vi "Mod בחירת בדיקות עבור הממסר.vi"(0 "Enable":bool=TRUE, 5 "error in (no error)":errorcluster) -> (11 "בחר הכל":bool, 12 "בדיקת מפל מתח בין דקי הממסר תחת עומס":bool, 13 "בדיקת זמן ניתוק הממסר":bool, 14 "בדיקת זמן מיתוג הממסר":bool, 15 "בדיקת צריכת זרם של סליל הפיקוד":bool, 16 "בדיקת מתח שחרור של סליל פיקוד ללא עומס":bool, 17 "בדיקת מתח תפיסה של סליל פיקוד ללא עומס":bool, 18 "OK":bool, 19 "error out":errorcluster)   [LabVIEW 2014]
doc: "Displays a standard dialog box that prompts users to enter information, such as a user name and password.\n--------------------\n\nThis Express VI is configured as follows:\n\nMessage to Display to the User:15A בחירת בדיקות עבור הממסר\nThe inputs are: \nCheckbox: בדיקת מתח תפיסה של סליל פיקוד ללא עומס\nCheckbox: בדיקת מתח שחרור של סליל פיקוד ללא עומס\nCheckbox: בדיקת צריכת זרם של סליל הפיקוד\nCheckbox: בדיקת זמן מיתוג הממסר\nCheckbox: בדיקת זמן ניתוק הממסר\nCheckbox: בדיקת מפל מתח בין דקי הממסר תחת עומס\nCheckbox: בחר הכל"
panel:
  in  "בחר הכל":bool
  in  "בדיקת מפל מתח בין דקי הממסר תחת עומס":bool
  in  "בדיקת זמן ניתוק הממסר":bool
  in  "בדיקת זמן מיתוג הממסר":bool
  in  "בדיקת צריכת זרם של סליל הפיקוד":bool
  in  "בדיקת מתח שחרור של סליל פיקוד ללא עומס":bool
  in  "בדיקת מתח תפיסה של סליל פיקוד ללא עומס":bool
  out "String":string="15A בחירת בדיקות עבור הממסר"
  in  "Cancel":bool
  in  "OK2":bool
  in  "OK1":bool
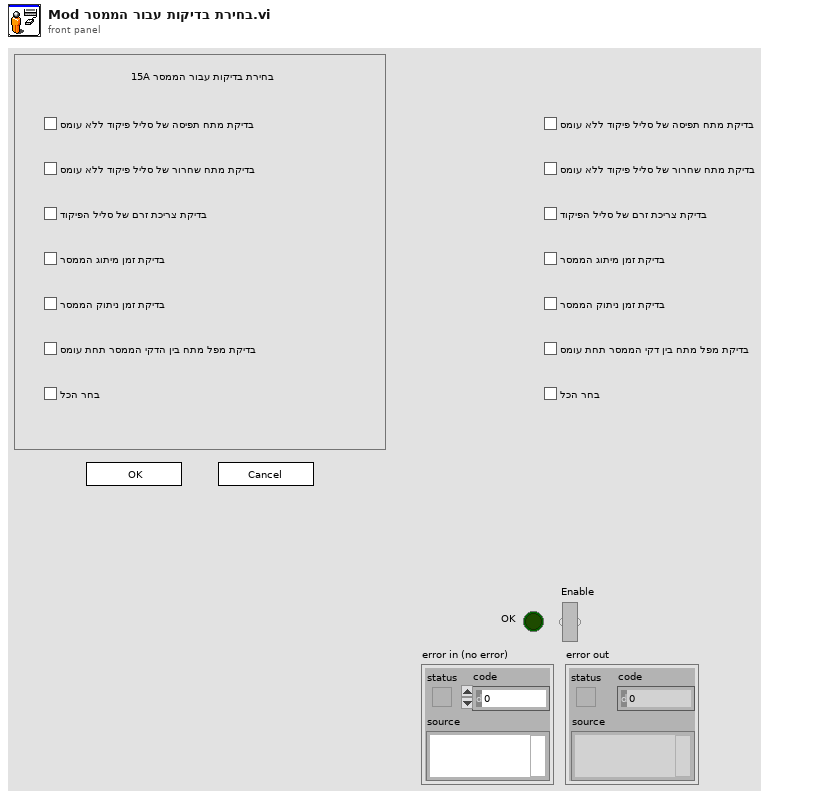
[diagram p1: front panel]
types:
  T1 = cluster{"Input Name":string, "Input Data Type":i32}[]
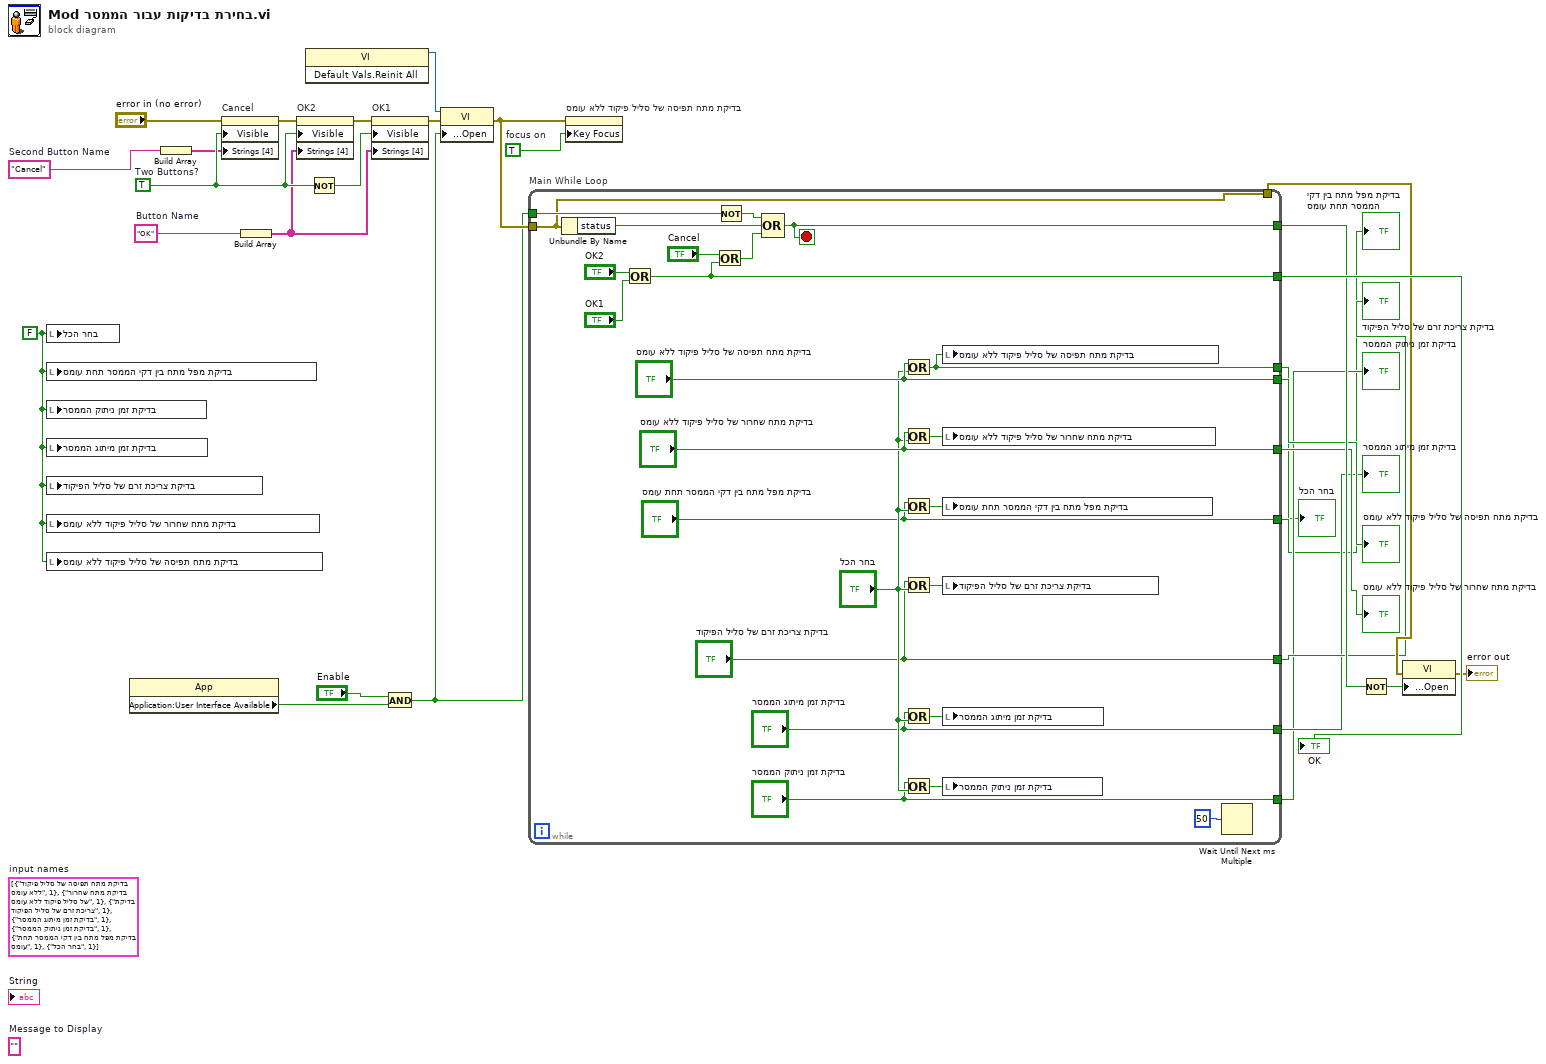
[diagram p0: block diagram]
diagram:
  w1 = FALSE ("בחר הכל")
  w8 = TRUE  # focus on
  (unwired) T1 [{"Input Name"="בדיקת מתח תפיסה של סליל פיקוד ללא עומס", "Input Data Type"=1}, {"Input Name"="בדיקת מתח שחרור של סליל פיקוד ללא עומס", "Input Data Type"=1}, {"Input Name"="בדיקת צריכת זרם של סליל הפיקוד", "Input Data Type"=1}, {"Input Name"="בדיקת זמן מיתוג הממסר", "Input Data Type"=1}, {"Input Name"="בדיקת זמן ניתוק הממסר", "Input Data Type"=1}, {"Input Name"="בדיקת מפל מתח בין דקי הממסר תחת עומס", "Input Data Type"=1}, {"Input Name"="בחר הכל", "Input Data Type"=1}]  # input names
  w21 = "Cancel"  # Second Button Name
  w19 = "OK"  # Button Name
  (unwired) ""  # Message to Display
  w29 = TRUE  # Two Buttons?
  n1 = local write "בחר הכל"(w1) -> ()
  n2 = local write "בדיקת מפל מתח בין דקי הממסר תחת עומס"(w1) -> ()
  n3 = local write "בדיקת זמן ניתוק הממסר"(w1) -> ()
  n4 = local write "בדיקת זמן מיתוג הממסר"(w1) -> ()
  n5 = local write "בדיקת צריכת זרם של סליל הפיקוד"(w1) -> ()
  n6 = local write "בדיקת מתח שחרור של סליל פיקוד ללא עומס"(w1) -> ()
  n7 = local write "בדיקת מתח תפיסה של סליל פיקוד ללא עומס"(w1) -> ()
  n8 = property class="App"() -> ("Application:User Interface Available"=w11:bool)  [unwired: 2 in, 2 out]
  n9 = Build Array(w21) -> (w22:string[])
  n10 = property on="Cancel" class="Bool"(error in="error in (no error)", "Visible"=w29, "Strings [4]"=w22) -> (error out=w26:errorcluster)  [unwired: 1 in, 1 out]
  n11 = Build Array(w19) -> (w20:string[])
  n12 = property on="OK2" class="Bool"(error in=w26, "Visible"=w29, "Strings [4]"=w20) -> (error out=w25:errorcluster)  [unwired: 1 in, 1 out]
  n13 = invoke class="VI" method="Default Vals.Reinit All"() -> (reference out=w10:refnum<vi>)  [unwired: 3 in, 2 out]
  n14 = Not(x=w29) -> (.not. x?=w27:bool)
  n15 = property on="OK1" class="Bool"(error in=w25, "Visible"=w27, "Strings [4]"=w20) -> (error out=w18:errorcluster)  [unwired: 1 in, 1 out]
  n16 = And(x="Enable", y=w11) -> (x .and. y?=w12:bool)
  n17 = property class="VI"(reference=w10, error in=w18, "Front Panel Window:Open"=w12) -> (error out=w17:errorcluster)  [unwired: 1 out]
  n18 = while "Main While Loop" {
    tunnel: [w50] -> w28
    tunnel: w12 -> [w48]
    tunnel: [w46] -> w23
    tunnel: w17 -> [w45]
    tunnel: [w45] -> w15
    tunnel: ["בדיקת מתח תפיסה של סליל פיקוד ללא עומס"] -> w9
    tunnel: ["בדיקת מתח שחרור של סליל פיקוד ללא עומס"] -> w7
    tunnel: ["בדיקת צריכת זרם של סליל הפיקוד"] -> w6
    tunnel: ["בדיקת זמן מיתוג הממסר"] -> w5
    tunnel: ["בדיקת זמן ניתוק הממסר"] -> w4
    tunnel: ["בדיקת מפל מתח בין דקי הממסר תחת עומס"] -> w3
    tunnel: [w42] -> w2
    stop <- w46 stop-if-true
    n19 = Unbundle By Name(w45) -> ("status"=w43:bool)
    n20 = Or(x="OK2", y="OK1") -> (x .or. y?=w50:bool)
    n21 = Or(x="Cancel", y=w50) -> (x .or. y?=w44:bool)
    n22 = Not(x=w48) -> (.not. x?=w47:bool)
    n23 = Compound Arithmetic op=OR(w47, w43, w44) -> (w46:bool)
    n24 = Or(x="בדיקת מתח תפיסה של סליל פיקוד ללא עומס", y="בחר הכל") -> (x .or. y?=w42:bool)
    n25 = Or(x="בדיקת מתח שחרור של סליל פיקוד ללא עומס", y="בחר הכל") -> (x .or. y?=w39:bool)
    n26 = Or(x="בדיקת מפל מתח בין דקי הממסר תחת עומס", y="בחר הכל") -> (x .or. y?=w33:bool)
    n27 = Or(x="בדיקת צריכת זרם של סליל הפיקוד", y="בחר הכל") -> (x .or. y?=w32:bool)
    n28 = Or(x="בדיקת זמן מיתוג הממסר", y="בחר הכל") -> (x .or. y?=w34:bool)
    n29 = Or(x="בדיקת זמן ניתוק הממסר", y="בחר הכל") -> (x .or. y?=w30:bool)
    n30 = local write "בדיקת מתח תפיסה של סליל פיקוד ללא עומס"(w42) -> ()
    n31 = local write "בדיקת מתח שחרור של סליל פיקוד ללא עומס"(w39) -> ()
    n32 = local write "בדיקת מפל מתח בין דקי הממסר תחת עומס"(w33) -> ()
    n33 = local write "בדיקת צריכת זרם של סליל הפיקוד"(w32) -> ()
    n34 = local write "בדיקת זמן מיתוג הממסר"(w34) -> ()
    n35 = local write "בדיקת זמן ניתוק הממסר"(w30) -> ()
    n36 = Wait Until Next ms Multiple(millisecond multiple=u32 50) -> ()  [unwired: 1 out]
  }
  "OK" <- w28
  "בדיקת מתח תפיסה של סליל פיקוד ללא עומס" <- w9
  "בדיקת מתח שחרור של סליל פיקוד ללא עומס" <- w7
  "בדיקת צריכת זרם של סליל הפיקוד" <- w6
  "בדיקת זמן מיתוג הממסר" <- w5
  "בדיקת זמן ניתוק הממסר" <- w4
  "בדיקת מפל מתח בין דקי הממסר תחת עומס" <- w3
  "בחר הכל" <- w2
  n37 = property on="בדיקת מתח תפיסה של סליל פיקוד ללא עומס" class="Bool (strict)"(error in=w17, "Key Focus"=w8) -> ()  [unwired: 1 in, 2 out]
  n38 = Not(x=w23) -> (.not. x?=w24:bool)
  n39 = property class="VI"(error in=w15, "Front Panel Window:Open"=w24) -> (error out=→"error out":errorcluster)  [unwired: 1 in, 1 out]
